vi "Danfysik Reset.vi"(8 "error in":errorcluster, 11 "cRIO I/O Device":refnum<k21>="Mod7\\Port2") -> (0 "error out":errorcluster)   [LabVIEW 2016]
uses:
  <vilib>/rvi/eio/common/nirviEmuTemplateMethod_errors.vi
  <vilib>/eio/EIOMethodNode/EIOMethodNode.xnode
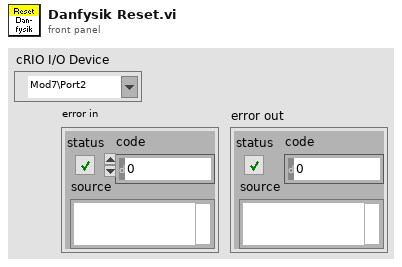
[diagram p1: front panel]
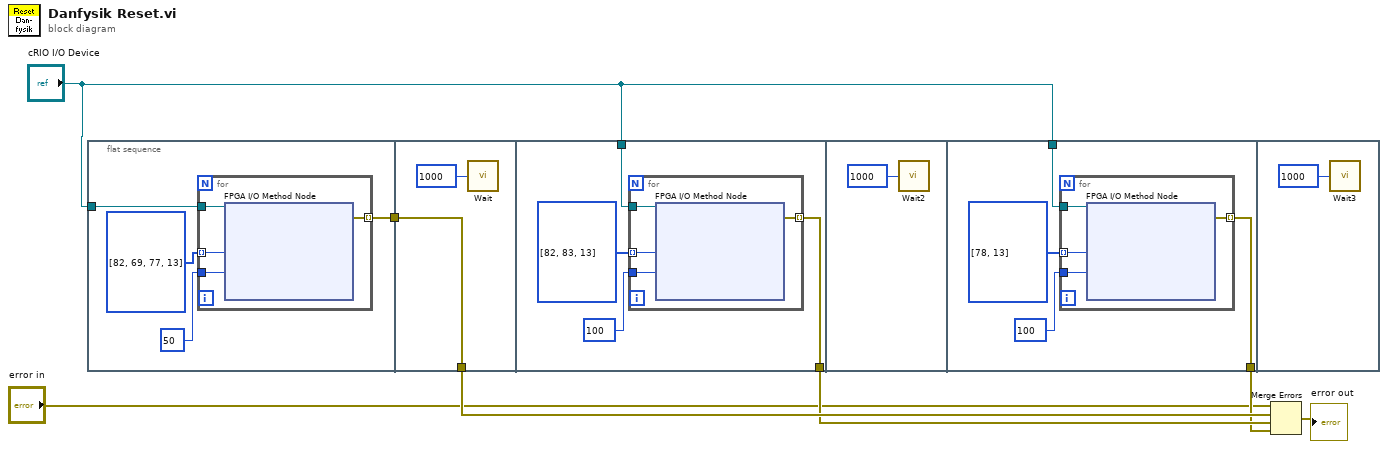
[diagram p0: block diagram]
diagram:
  n1 = flat-sequence {
    tunnel: "cRIO I/O Device" -> [w9]
    tunnel: [w8] -> w5
    tunnel: [w16] -> w6
    tunnel: w5 -> [w16]
    tunnel: "cRIO I/O Device" -> [w19]
    tunnel: [w18] -> w4
    tunnel: "cRIO I/O Device" -> [w28]
    tunnel: [w27] -> w3
    frame #0 {
      n2 = for {
        tunnel: 50 ("Timeout (ms)") -> [w14]
        tunnel: u8[] [82, 69, 77, 13] ("magnet ps") -> [w15] mode=indexing
        tunnel: w9 -> [w13]
        tunnel: [w12] -> w8 mode=indexing
        n3 = xnode "FPGA I/O Method Node"("FPGA I/O In"=w13, "Data"=w15, "Timeout (ms)"=w14) -> ("error out"=w12:errorcluster)  [unwired: 1 in, 2 out]
      }
    }
    frame #1 {
      n4 = call "Wait"("Count(mSec)"=u32 1000) -> ()  [unwired: 1 out]
    }
    frame #2 {
      n5 = for {
        tunnel: 100 ("Timeout (ms)") -> [w24]
        tunnel: u8[] [82, 83, 13] ("magnet ps") -> [w25] mode=indexing
        tunnel: w19 -> [w23]
        tunnel: [w22] -> w18 mode=indexing
        n6 = xnode "FPGA I/O Method Node"("FPGA I/O In"=w23, "Data"=w25, "Timeout (ms)"=w24) -> ("error out"=w22:errorcluster)  [unwired: 1 in, 2 out]
      }
    }
    frame #3 {
      n7 = call "Wait2"("Count(mSec)"=u32 1000) -> ()  [unwired: 1 out]
    }
    frame #4 {
      n8 = for {
        tunnel: 100 ("Timeout (ms)") -> [w32]
        tunnel: u8[] [78, 13] ("magnet ps") -> [w33] mode=indexing
        tunnel: w28 -> [w34]
        tunnel: [w31] -> w27 mode=indexing
        n9 = xnode "FPGA I/O Method Node"("FPGA I/O In"=w34, "Data"=w33, "Timeout (ms)"=w32) -> ("error out"=w31:errorcluster)  [unwired: 1 in, 2 out]
      }
    }
    frame #5 {
      n10 = call "Wait3"("Count(mSec)"=u32 1000) -> ()  [unwired: 1 out]
    }
  }
  n11 = Merge Errors("error in", w6, w4, w3) -> (→"error out":errorcluster)
